vi "PXI-Create Tasks.vi"(0 "I/O Channels":T2[](array[typedef]) {"Terminal configuration" items=["Default"=-1, "RSE"=10083, "Differential"=10106, "Pseudodifferential"=12529]}, 11 "error in (no error)":errorcluster) -> (4 "Task Specification Array":T1[](array[typedef]) {"Channels"."Terminal configuration" items=["Default"=-1, "RSE"=10083, "Differential"=10106, "Pseudodifferential"=12529]}, 15 "error out":errorcluster)   [LabVIEW 2020]
doc: "Creates (at most) one AO and one AI task per board. Loops through channels and decodes device and \"direction\" (i.e. AO or AI) for each channel. Creates a new task if device and direction have not been used. Otherwise, adds current channel to existing task."
uses:
  Type Defs/Channel Struct.ctl
  Type Defs/Task Specification Struct.ctl
  PXI Globals.vi
panel:
  in  "Dummy":T1 {"Channels"."Terminal configuration" items=["Default"=-1, "RSE"=10083, "Differential"=10106, "Pseudodifferential"=12529]}
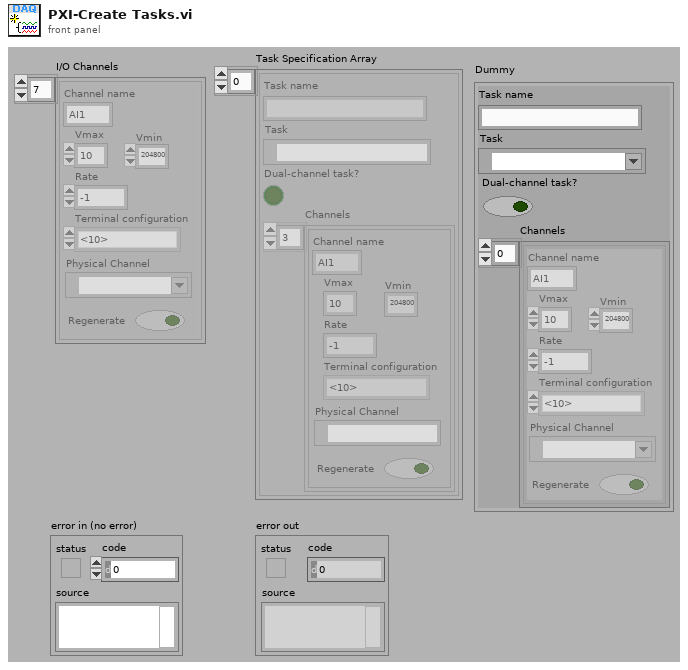
[diagram p1: front panel]
types:
  T1 = typedef "Task Specification Struct.ctl" = cluster{"Task name":string, "Task":refnum<k21>, "Dual-channel task?":bool, "Channels":T2[]}
  T2 = typedef "Channel Struct.ctl" = cluster{"Channel name":string, "Vmax":dbl, "Vmin":dbl, "Rate":dbl, "Terminal configuration":i32, "Physical Channel":tag, "Regenerate":bool}
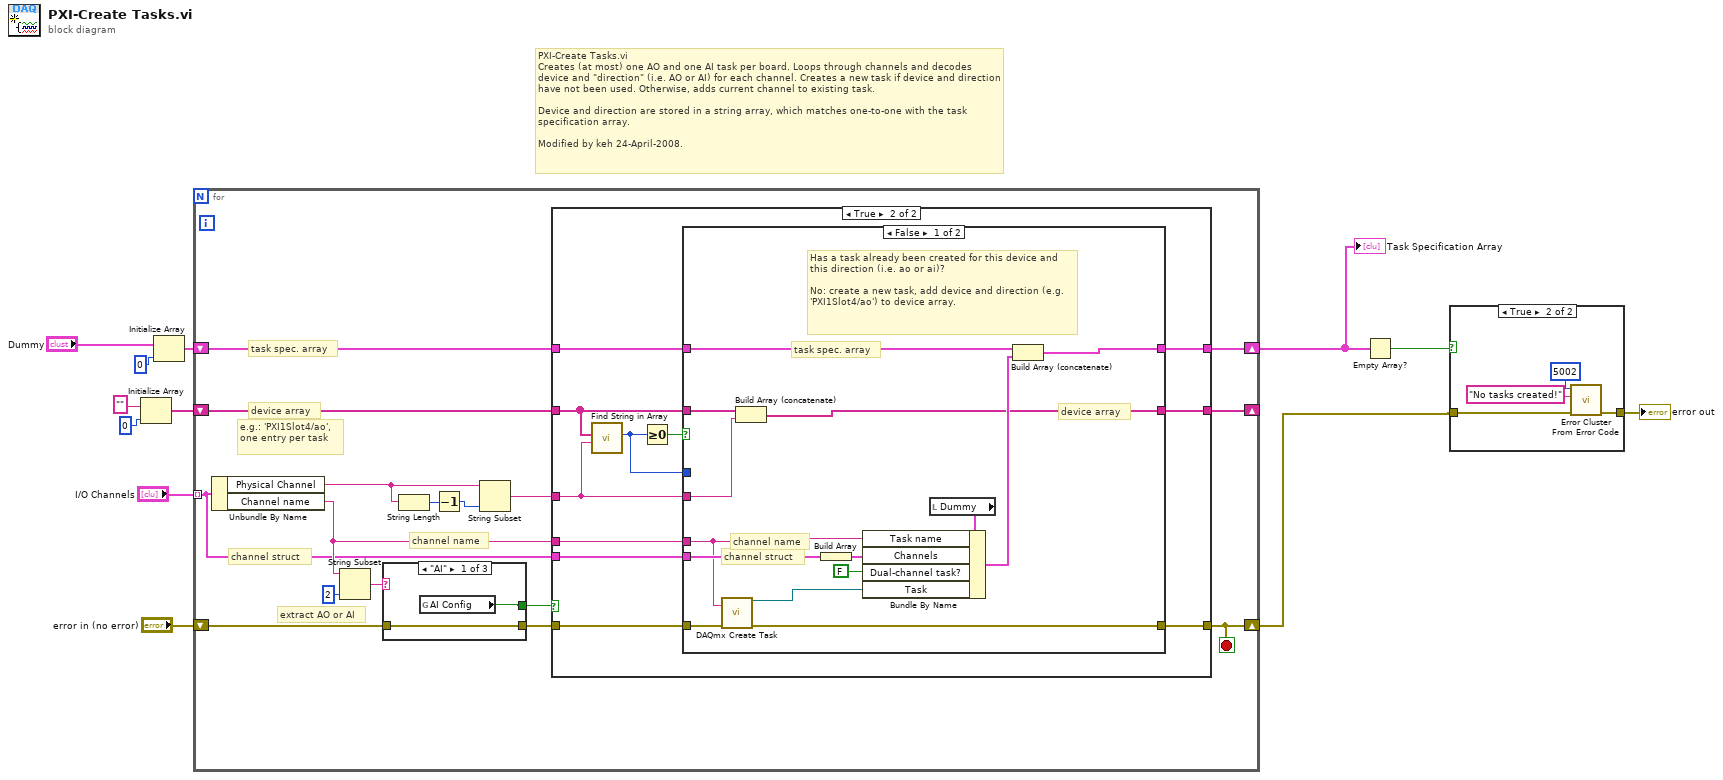
[diagram p0: block diagram]
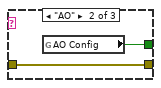
[diagram p3: hidden frame]
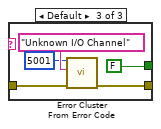
[diagram p4: hidden frame]
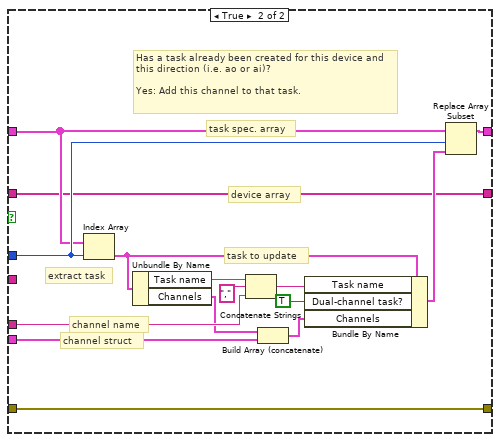
[diagram p6: hidden frame]
diagram:
  # "PXI-Create Tasks.vi\nCreates (at most) one AO and one AI task per board. Loops through channels and decodes device and \"direction\" (i.e. AO or AI) for each channel. Creates a new task if device and direction have not been used. Otherwise, adds current channel to existing task.\n\nDevice and direction are stored in a string array, which matches one-to-one with the task specification array.\n\nModified by keh 24-April-2008."
  n1 = Initialize Array("", 0 ("dimension size")) -> (w4:string[])
  n2 = Initialize Array("Dummy", 0 ("dimension size")) -> (w10:T1[])
  n3 = for {
    tunnel: "I/O Channels" -> [w17] mode=indexing
    shift-right: [w27] -> w2
    shift-left: w10 -> [w28]
    shift-right: [w13] -> w3
    shift-left: "error in (no error)" -> [w26]
    shift-right: [w18] -> _
    shift-left: w4 -> [w20]
    stop <- w13 stop-if-true
    # "channel struct"
    # "channel name"
    # "task spec. array"
    # "e.g.: 'PXI1Slot4/ao',\none entry per task"
    # "device array"
    # "extract AO or AI"
    n4 = Unbundle By Name(w17) -> ("Physical Channel"=w14:tag, "Channel name"=w19:string)
    n5 = String Subset(string=w19, length (rest)=2 ("length (rest)")) -> (substring=w24:string)  [unwired: 1 in]
    n6 = case shown="\"AI\"" w24 {
      tunnel: w26 -> [w30 w32 w35]
      tunnel: [w30 w32 w34] -> w23
      tunnel: [w29 w31 FALSE] -> w22
      frame "AI" {
        n7 = global read "PXI Globals.vi" "AI Config"() -> (w29:bool)
      }
      frame "AO" {
        n8 = global read "PXI Globals.vi" "AO Config"() -> (w31:bool)
      }
      frame Default {
        n9 = call <vilib>:"Error Cluster From Error Code.vi"("error in (no error)"=w35, "error message (\"\")"="Unknown I/O Channel" ("error message (\"\")"), "error code (0)"=5001) -> ("error out"=w34:errorcluster)  [unwired: 6 in]
      }
    }
    n10 = String Length(string=w14) -> (length=w16:i32)
    n11 = Decrement(x=w16) -> (x-1=w15:i32)
    n12 = String Subset(string=w14, length (rest)=w15) -> (substring=w21:string)  [unwired: 1 in]
    n13 = case shown="True" w22 {
      tunnel: [w40 w43] -> w27
      tunnel: w28 -> [w40 w44]
      tunnel: w23 -> [w39 w50]
      tunnel: [w39 w45] -> w13
      tunnel: w21 -> [_ w46]
      tunnel: w20 -> [w38 w47]
      tunnel: w19 -> [_ w49]
      tunnel: [w38 w42] -> w18
      tunnel: w17 -> [_ w41]
      frame False {
      }
      frame True {
        n14 = call "Find String in Array.vi"("String"=w46, "Array"=w47) -> ("Index"=w48:i32)  [unwired: 9 in]
        n15 = Greater Or Equal To 0?(x=w48) -> (x >= 0?=w51:bool)
        n16 = case shown="False" w51 {
          tunnel: w50 -> [w65 w66]
          tunnel: w49 -> [w52 w73]
          tunnel: w48 -> [_ w79]
          tunnel: w47 -> [w57 w70]
          tunnel: w46 -> [w56 _]
          tunnel: [w63 w66] -> w45
          tunnel: w44 -> [w60 w78]
          tunnel: [w59 w76] -> w43
          tunnel: [w55 w70] -> w42
          tunnel: w41 -> [w58 w67]
          frame False {
            # "channel name"
            # "channel struct"
            # "task spec. array"
            # "Has a task already been created for this device and this direction (i.e. ao or ai)?\n\nNo: create a new task, add device and direction (e.g. 'PXI1Slot4/ao') to device array."
            # "device array"
            n17 = call <vilib>:"DAQmx Create Task.vi"("new task name"=w52, "error in"=w65) -> ("task out"=w53:refnum<k21>, "error out"=w63:errorcluster)  [unwired: 12 in]
            n18 = Build Array (concatenate)(w57, w56) -> (w55:string[])
            n19 = Build Array(w58) -> (w54:T2[])
            n20 = local read "Dummy"() -> (w62:T1)
            n21 = Bundle By Name(cluster=w62, "Task name"=w52, "Channels"=w54, "Dual-channel task?"=FALSE, "Task"=w53) -> (w61:T1)
            n22 = Build Array (concatenate)(w60, w61) -> (w59:T1[])
          }
          frame True {
            # "task to update"
            # "channel name"
            # "channel struct"
            # "extract task"
            # "device array"
            # "task spec. array"
            # "Has a task already been created for this device and this direction (i.e. ao or ai)?\n\nYes: Add this channel to that task."
            n23 = Index Array(array=w78, index=w79) -> (element=w80:T1)
            n24 = Unbundle By Name(w80) -> ("Task name"=w75:string, "Channels"=w69:T2[])
            n25 = Concatenate Strings(w75, "," ("string"), w73) -> (w72:string)
            n26 = Build Array (concatenate)(w69, w67) -> (w68:T2[])
            n27 = Bundle By Name(cluster=w80, "Task name"=w72, "Dual-channel task?"=TRUE, "Channels"=w68) -> (w77:T1)
            n28 = Replace Array Subset(array=w78, new element=w77, index=w79) -> (w76:T1[])
          }
        }
      }
    }
  }
  "Task Specification Array" <- w2
  n29 = Empty Array?(array=w2) -> (empty?=w1:bool)
  n30 = case shown="True" w1 {
    tunnel: w3 -> [w81 w83]
    tunnel: [w81 w82] -> w7
    frame False {
    }
    frame True {
      n31 = call <vilib>:"Error Cluster From Error Code.vi"("error in (no error)"=w83, "error message (\"\")"="No tasks created!" ("error message (\"\")"), "error code (0)"=5002) -> ("error out"=w82:errorcluster)  [unwired: 6 in]
    }
  }
  "error out" <- w7
